vi "MTM2_putSample_mirrorPositionMeasured.vi"(8 "error in (no error)":errorcluster, 11 "mirrorPositionMeasured_Ctl":T1) -> (0 "error out":errorcluster, 2 "function return":i32, 3 "mirrorPositionMeasured_Ctl out":T1)   [LabVIEW 2018, in "SALLV_MTM2.lvlib"]
doc: "int MTM2_shm_putSample_mirrorPositionMeasuredLV(MTM2_mirrorPositionMeasuredLV *mirrorPositionMeasured_Ctl );"
uses:
  SALLV_MTM2.lvlib
  DataTypes/mirrorPositionMeasured.ctl
  SALLV_MTM2.so
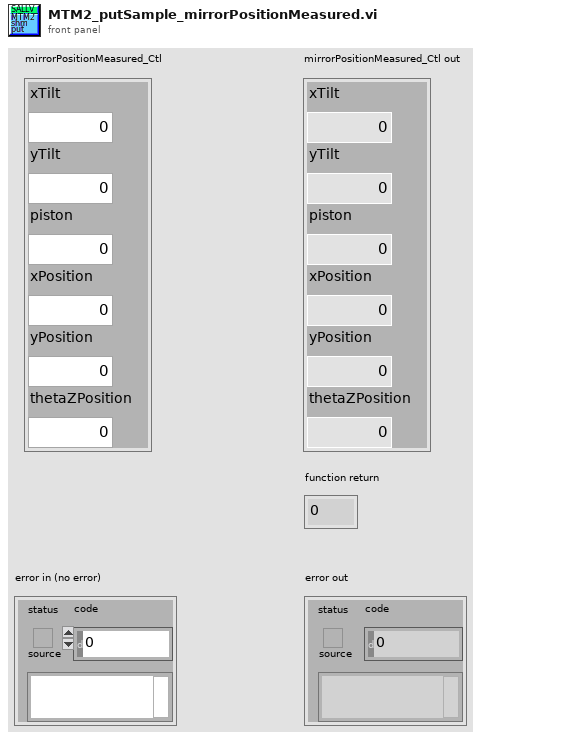
[diagram p1: front panel]
types:
  T1 = typedef "SALLV_MTM2.lvlib/mirrorPositionMeasured.ctl" = cluster{"xTilt":dbl, "yTilt":dbl, "piston":dbl, "xPosition":dbl, "yPosition":dbl, "thetaZPosition":dbl}
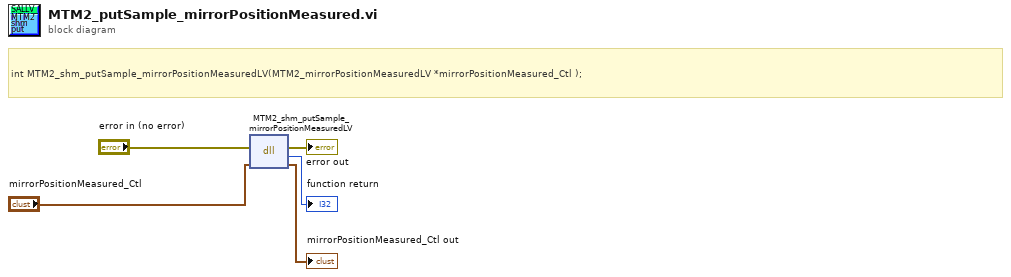
[diagram p0: block diagram]
diagram:
  # "int MTM2_shm_putSample_mirrorPositionMeasuredLV(MTM2_mirrorPositionMeasuredLV *mirrorPositionMeasured_Ctl );"
  n1 = dll-call lib="home/ttsai/Document/salApiMTM2/SALLV_MTM2/SALLV_MTM2.*" fn="MTM2_shm_putSample_mirrorPositionMeasuredLV"(error in="error in (no error)", "mirrorPositionMeasured_Ctl"="mirrorPositionMeasured_Ctl") -> (error out=→"error out":errorcluster, →"function return":i32, "mirrorPositionMeasured_Ctl"=→"mirrorPositionMeasured_Ctl out":T1)  [unwired: 2 in, 1 out]
